vi "Check if configuration files exist.vi"(8 "error in (no error)":errorcluster, 11 "AutofocusBase in":refnum<class "Autofocus.lvclass">) -> (0 "error out":errorcluster, 2 "configuration file exists?":bool, 3 "AutofocusBase out":refnum<class "Autofocus.lvclass">)   [LabVIEW 2012]
doc: "Checks whether all required configuration files for the component exist."
uses:
  Autofocus.lvclass
  <vilib>/Distrio/Murmex/Murmex/Murmex.lvclass
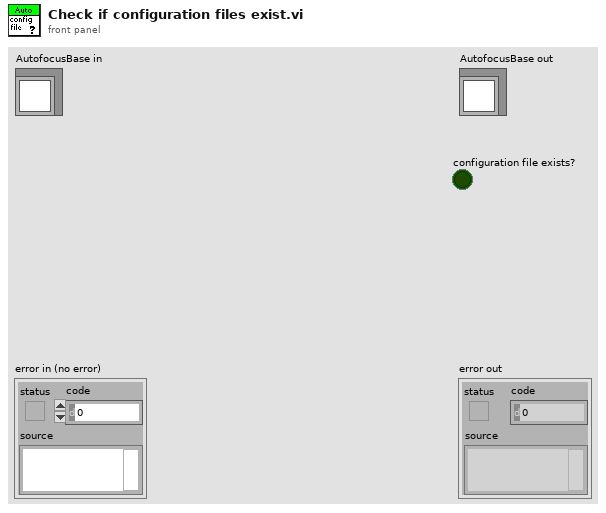
[diagram p1: front panel]
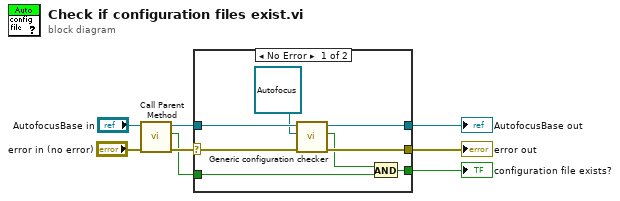
[diagram p0: block diagram]
diagram:
  n1 = call-parent "Call Parent Method"("error in (no error)"="error in (no error)", "MurmexBase in"="AutofocusBase in") -> ("error out"=w6:errorcluster, "configuration file exists?"=w4:bool, "MurmexBase out"=w2:refnum<class "Autofocus.lvclass">)  [unwired: 7 in]
  n2 = case shown="No Error" w6 {
    selector: w6 -> [w16 w18]
    tunnel: [w15 w18] -> w5
    tunnel: w4 -> [w14 w17]
    tunnel: [w12 w17] -> w3
    tunnel: w2 -> [w11 w19]
    tunnel: [w9 w19] -> w1
    frame No Error {
      n3 = call <vilib>:"Generic configuration checker.vi"("error in (no error)"=w16, 10:refnum<class "Autofocus.lvclass"> refnum ("Autofocus.lvclass"), "Murmex in"=w11) -> ("error out"=w15:errorcluster, "configuration file exists?"=w13:bool, "Murmex out"=w9:refnum<class "Autofocus.lvclass">)  [unwired: 6 in]
      n4 = And(x=w13, y=w14) -> (x .and. y?=w12:bool)
    }
    frame Error {
    }
  }
  "error out" <- w5
  "AutofocusBase out" <- w1
  "configuration file exists?" <- w3
